vi "AlliGator Overlay Phasor Ratio or Derived Quantity on Source Image v3.vi"(7 "Image Color Scale Information":T2, 8 "Error In":errorcluster, 10 "Source Image Display":T1, 11 "AlliGator IV DVR in":refnum<data-value>) -> (0 "Error Out":errorcluster, 1 "# Overlay Pixels":i32, 2 "Source Image Display out":T1, 3 "AlliGator IV DVR out":refnum<data-value>)   [LabVIEW 2021, in "AlliGator Phasor Plot.lvlib"]
doc: "Computes and overlays the phasor ratio map (or map of a derived quantity) on the Source Image."
uses:
  AlliGator Phasor Plot.lvlib
  <vilib>/vision/Image Controls.llb/IMAQ Image.ctl
  Internal Variables/AlliGator Internal Variables v2.ctl
  Internal Variables/AlliGator Gate Image Set.ctl
  Files/AlliGator FLI Dataset Type.ctl
  Files/AlliGator Data Series Type.ctl
  Dual-Channel Datasets/AlliGator Dataset Channel.ctl
  Settings/AlliGator Gate Arithmetic.ctl
  Source Image/AlliGator Displayed Image.ctl
  Image/Named ROI Description.ctl
  Phasor Graph/AlliGator Decay Metadata v3.ctl
  Decay Analysis/Decay Preprocessing/AlliGator Decay Background Subtraction Info.ctl
  Decay Analysis/Decay Preprocessing/AlliGator Baseline Subtraction Method.ctl
  Graphs/XY Graph/XY Graph Plot Shift Parameters.ctl
  Graphs/XY Graph/XY Graph Plot Shift Method.ctl
  Decay Analysis/Decay Preprocessing/AlliGator Decay Extrapolation Parameters.ctl
  Phasor/Calibration Phasor (m, phi).ctl
  Phasor/Phasor Reference Series.ctl
  Phasor/Phasor Calibration Map v2.ctl
  Phasor/Phasor (g, s).ctl
  Phasor Graph/AlliGator Raw Phasor Plot Data v4.ctl
  Phasor/Phasor Standard Deviation Options.ctl
  AlliGator Phasor Multi-Harmonic Data.ctl
  Phasor/Phasor Harmonic Data.ctl
  Decay Fit Parameter Map/AlliGator Decay Fit Options & Parameters v2.ctl
  Fits/IRF(X)PSED/Decay Fit Options v2.ctl
  Fits/Decay Convolution/Decay Model.ctl
  Fits/Residual Type.ctl
  Fits/IRF(X)PSED/Fit Weights Type.ctl
  Fits/Non-linear Fitting Method v2.ctl
  Fits/Fit Calculation Method.ctl
  Fits/Non-linear Fitting Algorithm.ctl
  Decay Analysis/Decay Fit/AlliGator Decay Fit Parameter Constraints 2.ctl
  Fits/IRF(X)PSED/Decay Fit Parameters In List.ctl
  Fits/IRF(X)PSED/MLE Baseline Offset Type.ctl
  Decay Analysis/Decay Preprocessing/AlliGator Decay Preprocessing Parameters.ctl
  Fits/IRF(X)PSED/Decay Fit Parameters & Derived Quantities List v2.ctl
  Decay Fit Parameter Map/AlliGator Parameter Maps Data.ctl
  Image/Image Color Scale Information.ctl
  Settings/AlliGator Settings List.ctl
  Palette/Image Palette Information.ctl
  Image/Image Display Palette Type.ctl
  Globals, Variables, Constants/AlliGator Variables List.ctl
  Phasor Ratio/AlliGator Phasor Ratio Data.ctl
  Phasor Ratio/AlliGator Phasor Ratio Color-Coded Quantity.ctl
  Phasor/Phasor Ratio Type.ctl
  Settings/AlliGator Partial Data Information.ctl
  Palette/Limit+NaN Colors.ctl
  Variant/Variant to Data/Variant to DBL.vi
  Variant/Variant to Data/Variant to Boolean.vi
  Variant/Variant to Data/Variant to String.vi
  Variant/Variant to Data/Variant to U32.vi
  <vilib>/vision/NI_Vision_Development_Module.lvlib
  Settings/AlliGator Settings.lvlib
  Variant/Variant to Data/Variant to Data.lvlib
  Image/Image.lvlib
  Palette/Palette.lvlib
  Globals, Variables, Constants/AlliGator Globals, Variables & Constants.lvlib
  Phasor Ratio/AlliGator Phasor Ratio.lvlib
  Time/Time.lvlib
  Error/Error.lvlib
  Phasor/Phasor.lvlib
  Utilities/Utilities.lvlib
  Decay Analysis/Decay Preprocessing/AlliGator Decay Preprocessing.lvlib
  Graphs/XY Graph/XY Graph Add-Ons.lvlib
  Phasor Graph/AlliGator Phasor Graph.lvlib
  Files/AlliGator Files.lvlib
  Source Image/AlliGator Source Image.lvlib
  Internal Variables/AlliGator Internal Variables.lvlib
  Fits/Fits.lvlib
  Decay Analysis/Decay Fit/AlliGator Decay Fit.lvlib
  Decay Fit Parameter Map/AlliGator Decay Fit Parameter Map.lvlib
  Dual-Channel Datasets/AlliGator Dual-Channel Datasets.lvlib
panel:
  out "Overlay Copy (s)":dbl
  out "Overlay Erase (s)":dbl
  out "Overlay Compute (s)":dbl
  # "see the AlliGator License on the block diagram (Ctrl+E or Window:Show Block Diagram)"
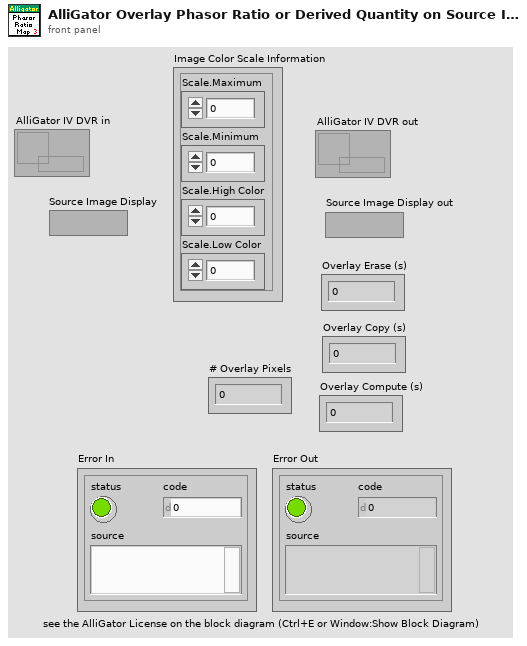
[diagram p1: front panel]
types:
  T1 = typedef "IMAQ Image.ctl" = refnum<image>
  T2 = typedef "Image.lvlib/Image Color Scale Information.ctl" = cluster{"Scale.Maximum":dbl, "Scale.Minimum":dbl, "Scale.High Color":u32, "Scale.Low Color":u32}
  T3 = typedef "Palette.lvlib/Limit+NaN Colors.ctl" = cluster{"Color Scale High Color":cluster{"Red (or Hue) value":u8, "Green (or Sat) value":u8, "Blue (or Light or Val) value":u8}, "Color Scale Low Color":cluster{"Red (or Hue) value":u8, "Green (or Sat) value":u8, "Blue (or Light or Val) value":u8}, "NaN Color":cluster{"Red (or Hue) value":u8, "Green (or Sat) value":u8, "Blue (or Light or Val) value":u8}}
  T4 = typedef "AlliGator Settings.lvlib/AlliGator Settings List.ctl" = enum16{"GUI:Visible Settings Tab", "GUI:Last Run Version", "Source Image:Use Image Histogram for Contrast", "Source Image:Low Count Pixels Rejection Options", "Source Image:High Count Pixels Rejection Options", "Source Image:Use Image Brightness", "Source Image:Blend Overlay with Image Background", "Source Image:Use Fixed ROI Diameter", "Source Image:ROI Diameter", "Source Image:ROI Center Color", "Source Image:Peak Threshold", "Source Image:Intensity Threshold", "Source Image:Image Binning Options", "Source Image:Image Smoothing Options", "Source Image:Image Histogram Active", "Source Image:Invert Binary Mask", "Source Image:Hot Pixel Removal", "Source Image:Overlay Analyzed ROI Center", "Source Image:Auto-Adjust Contrast", "Source Image:Histogram Lower Percentile", "Source Image:Histogram Upper Percentile", "Source Image:Save Source Image", "Source Image:Scale Bar Options", "Source Image:Image Resolution (Pixel Size)", "Source Image:Flatfield Correction", "Source Image:Show Dead Left Columns Correction", "Source Image:Dead Left Columns Correction", "Source Image:Image Pre-Processing Operations Order", "Source Image:Overlay ROI Median", "Source Image:Median Overlay Color", "Data Information:Gate Width", "Data Information:Nanotime Gate Separation", "Data Information:Macrotime Gate Separation", "Data Information:Gate Step", "Data Information:# Gates", "Data Information:Gate Image Exposure", "Data Information:Gate Image Integration", "Data Information:Gates to Skip", "Data Information:Gates to Keep", "Data Information:Define Gates to", "Data Information:Channel Name", "Data Information:Available Channel Names", "Data Information:Channel Arithmetic", "Data Information:Background File Subtraction", "Data Information:Background File", "Data Information:Background Scaling Factor", "Data Information:Background Pile-up Correction", "Data Information:Background Pixel Well Capacity", "Data Information:Laser Period", "Data Information:SYNC Period", "Data Information:Pile-up Correction", "Data Information:Pixel Well Capacity", "Data Information:Dataset Scaling Factor", "Fluorescence Decay_Decay Pre-Processing:Reverse Gates", "Fluorescence Decay_Decay Pre-Processing:Verbose Decay Pre-Processing", "Fluorescence Decay_Decay Pre-Processing:Use Decay Pre-Processing", "Fluorescence Decay_Decay Pre-Processing:Background Subtraction", "Fluorescence Decay_Decay Pre-Processing:Background Definition Range", "Fluorescence Decay_Decay Pre-Processing:Baseline Subtraction Method", "Fluorescence Decay_Decay Pre-Processing:Decay Pre-Processing Operations Order", "Fluorescence Decay_Decay Pre-Processing:Smoothing Parameter", "Fluorescence Decay_Decay Pre-Processing:Shift Decay", "Fluorescence Decay_Decay Pre-Processing:Decay Shift Parameters", "Fluorescence Decay_Decay Pre-Processing:Fold Decay", "Fluorescence Decay_Decay Pre-Processing:# Folds", "Fluorescence Decay_Decay Pre-Processing:1-Normalize Decay", "Fluorescence Decay_Decay Pre-Processing:[0-1]-Normalize Decay", "Fluorescence Decay_Decay Pre-Processing:Smoothen Decay", "Fluorescence Decay_Decay Pre-Processing:Extrapolate Decay", "Fluorescence Decay_Decay Pre-Processing:Use Periodicity", "Fluorescence Decay_Decay Pre-Processing:Use Cursors", "Fluorescence Decay_Decay Pre-Processing:Tail Fraction", "Fluorescence Decay_Decay Pre-Processing:Head Fraction", "Fluorescence Decay_Decay Pre-Processing:Additional Points", "Fluorescence Decay_Decay Pre-Processing:Straighten Decay", "Fluorescence Decay_Decay Pre-Processing:Constant Background", "Fluorescence Decay_Decay Pre-Processing:Pixel-Normalize Decay", "Fluorescence Decay_Advanced Analysis:Extract IRF instead of Decay", "Fluorescence Decay_Advanced Analysis:IRF Extraction Options", "Fluorescence Decay_Advanced Analysis:IRF Optimization Options", "Fluorescence Decay_Advanced Analysis:Square Pulse Options", "Fluorescence Decay_Advanced Analysis:IRF Order", "Fluorescence Decay_Advanced Analysis:IRF Time Constants", "Fluorescence Decay_Advanced Analysis:Wavelet Analysis Options", "Fluorescence Decay_Advanced Analysis:Average Lifetime Options", "Fluorescence Decay_Fit Options:Fit Options", "Fluorescence Decay_Fit Options:Use Legacy Fitting Approach", "Fluorescence Decay_Fit Options:Use Data Information Laser Period", "Fluorescence Decay_Fit Parameters:Displayed Fit Parameters", "Fluorescence Decay_Fit Parameters:Fit Parameter Constraints", "Fluorescence Decay_Fit Parameters:Export Tabulated Results", "Fluorescence Decay_Fit Parameters:MLE Baseline Offset Type", "Fluorescence Decay_Fit Parameters:MLE Baseline Offset", "Fluorescence Decay_Fit Parameters:Guess Parameter Names", "Fluorescence Decay_Fit Parameters:Guess Parameter Values", "Fluorescence Decay_Fit Parameters:Guess Parameters Options", "Fluorescence Decay_Fit Parameters:Optimal Offset Selection Criterion", "Fluorescence Decay_Styles:Show Last Decay Only", "Fluorescence Decay_Styles:Decay Graph Color Array", "Fluorescence Decay:Decay Graph Active", "Fluorescence Decay Statistics:Min Peak Value", "Fluorescence Decay Statistics:Reject Low Decay Peak Pixels", "Fluorescence Decay Statistics:Reject High Decay Peak Pixels", "Fluorescence Decay Statistics:Max Peak Value", "Time Traces:Use File Timestamp", "Time Traces:Time Step", "Time Traces:Use Intensity Correction File", "Time Traces:Intensity Correction File", "Phasor Plot:Phasor Plot Smoothing Options", "Phasor Plot:Phasor Plot Size", "Phasor Plot:Phasor Plot Graphics Options", "Phasor Plot:Cumulative Phasor Plot", "Phasor Plot:Use Phasor Brightness", "Phasor Plot:Blend Overlay with Phasor Background", "Phasor Plot:Save Phasor Plot", "Phasor Plot:Show References", "Phasor Plot:Phasor Ratio Decay Range", "Phasor Plot:Exponential Fading", "Phasor Plot:Phasor Ratio Reference Colors", "Phasor Plot:Reference Radius", "Phasor Plot:Show Color Map Vertices", "Phasor Plot:Phasor Plot Active", "Phasor Plot:Phasor Ratio Color Map Type", "Phasor Plot:Phasor Ratio Color Map", "Phasor Plot:Phasor Ratio Display Range", "Phasor Plot:Selected Image ROI(s)", "Phasor Plot:All Image ROIs", "Phasor Plot:Selected Phasor Plot ROI(s)", "Phasor Plot:All Phasor Plot ROIs", "Phasor Plot:Phasor Ratio Color-Coded Quantity", "Phasor Plot:Store Phasor Harmonics", "Phasor Plot:Draw Reference Segment", "Phasor Plot:User-Defined Quantity", "Phasor Plot:Color Scale High Color", "Phasor Plot:Color Scale Low Color", "Phasor Graph:Phasor Frequency", "Phasor Graph:Phasor Ratio Type", "Phasor Graph:Pixel-level Phasor Computation", "Phasor Graph:Save Phasor Graph", "Phasor Graph:Phasor Graph Active", "Phasor Graph:Phasor SDV Options", "Phasor Calibration:Use Backup Calibration if needed", "Phasor Graph:Define Shortest Lifetime as", "Phasor Calibration:Backup Calibration Type", "Phasor Calibration:Calibration Type", "Phasor Calibration:Calibration Lifetime", "Phasor Calibration:Calibration Map Algorithm", "Single-Exponential Phasor Locus (SEPL):Gate Parameters", "Single-Exponential Phasor Locus (SEPL):User-defined Gate", "Single-Exponential Phasor Locus (SEPL):User-defined IRF", "Single-Exponential Phasor Locus (SEPL):Phasor Parameters", "Single-Exponential Phasor Locus (SEPL):Decay & IRF Parameters", "Single-Exponential Phasor Locus (SEPL):Display Parameters", "Lifetime Analysis:Decay Analysis Parameters", "Lifetime Analysis:Lifetime Map Active", "Plugins:Python Settings", "Miscellaneous:Verbose Mode", "Miscellaneous:Beep after Script", "Miscellaneous:Saved Image File Format", "Miscellaneous:Exported Gate Image Settings", "Miscellaneous:Include Loading in Timing", "Miscellaneous:Verbose Settings Mode", "Miscellaneous:Histogram Options", "Miscellaneous:Beep on Error", "Miscellaneous:# Logical Processors Used", "Miscellaneous:ROI Description Max Characters", "Miscellaneous:Verbose Error Mode", "Miscellaneous:Transparent Mask Color"}
  T5 = typedef "AlliGator Settings.lvlib/AlliGator Partial Data Information.ctl" = cluster{"Laser Period":dbl[unit], "SYNC Period":dbl[unit], "# Gates":u32, "Gate Separation":dbl[unit]}
  T6 = typedef "Phasor.lvlib/Phasor Ratio Type.ctl" = enum32{"Intensity-weighted", "Amplitude-weighted"}
  T7 = typedef "AlliGator Phasor Ratio.lvlib/AlliGator Phasor Ratio Color-Coded Quantity.ctl" = enum16{"Phasor Ratio (f1 or a1)", "Average Lifetime (<tau>_i or <tau>_a))", "User-Defined Quantity"}
  T8 = typedef "AlliGator Phasor Ratio.lvlib/AlliGator Phasor Ratio Data.ctl" = cluster{"Complex Phasor":csg, "Phasor Ratio":sgl, "z_1":csg, "z_2":csg, "Mapped Quantity":sgl}
  T9 = typedef "AlliGator Globals, Variables & Constants.lvlib/AlliGator Variables List.ctl" = enum16{"---- GUI ----", "GUI:Initialization Status", "GUI:State Indicators Refnum", "GUI:Original AlliGator Menu Items", "GUI:Current Action Loop State", "GUI:Script in progress", "GUI:Playback", "GUI:Loop Playback", "GUI:Search ROI Used", "GUI:Search ROI", "Decay Graph Max Legend Size", "Intensity Graph Max Legend Size", "Decay Statistics Graph Max Legend Size", "Phasor Graph Max Legend Size", "Phasor Ratio Graph Max Legend Size", "Lifetime Graph Max Legend Size", "---- Files ----", "Files:Export Dataset Frames as Individual Files", "Files:Show Batch Export Help Balloons", "Files:Frames in Dataset", "Files:ptu File Frame Start Indices", "Files:Current Frame in Dataset", "Files:Current Frame Timestamp", "Files:Dataset Loaded", "Files:Dataset Metadata", "Files:Dataset Channel", "Files:Dataset Data Description", "Files:Background Dataset Metadata", "Files:Background Dataset Channel", "Files:Background Dataset Data Description", "Files:Background File Subtraction", "Files:Background File Path", "Files:Background File Pile-up Correction", "Files:Background File Pixel Well Capacity", "Files:Background File Scaling Factor", "Files:Current Dataset Load Settings", "Files:Dataset Path", "Files:ICCD-specific Information", "Files:Macrotime Gate Separation", "------ Python Plugins ------", "Python Plugins:Information", "Python Plugins:Python Session", "Python Plugins:Valid Python Session?", "---- Source Image ----", "Source Image:ROIs", "Source Image:Current ROI", "Source Image:ROI Event Refnum", "X_Source Image:Display Range", "X_Source Image:Palette Information", "X_Source Image:Type of Displayed Image", "X_Time Gate Slider", "Source Image:Palette List", "Source Image:Scale", "Source Image:ROI Overlay Color", "Source Image:Overlay to Erase", "Source Image:Is Displayed Image Accumulated", "Source Image:White Light Image Modified", "Source Image:Mask Image Modified", "---- Image Profile Window ----", "Image Profile:Window Event Refnum", "Image Profile:IntensityType", "Image Profile:Intensity Average Type", "Image Profile:Intensity-weighted SDV", "Image Profile:Box Profile Type", "Image Profile:Window Open", "Image Profile:Plotted Fit Parameter", "------ Phasor Graph -------", "Phasor Graph:Show Line", "---- Phasor Plot ---", "Phasor Plot:Parameters Changed", "Phasor Plot:FLI Dataset Modified since last Calculation", "Phasor Harmonics Data", "Selected Phasor Harmonics", "Phasor Harmonic Manager Event Refnum", "Phasor Plot:ROIs", "Phasor Plot:Current ROI", "Phasor Plot:ROI Event Refnum", "Phasor Plot:Image Reference Points", "Phasor Plot:Computed", "Phasor Plot:Palette Information", "Phasor Plot:Palette List", "Phasor Plot:Phasor Ratio Palette Information", "Phasor Plot:Phasor Ratio Palette List", "Phasor Plot:Image Scale", "Phasor Plot:Image Overlay to Erase", "Phasor Plot:Image Elements to Update", "Phasor Plot:Current Calculation Parameters", "Phasor Plot:Current Calibration Options", "Phasor Plot:Reset Cumulated Phasor Plot", "Phasor Plot:Reference 1", "Phasor Plot:Lifetime Reference 1", "Phasor Plot:Reference 1 Frequency", "Phasor Plot:Reference 2", "Phasor Plot:Lifetime Reference 2", "Phasor Plot:Reference 2 Frequency", "---- Decay Analysis ----", "Number of Selected Decays to Fit", "LS Fit Results", "LAR Fit Results", "BS Fit Results", "Last Decay Max - Min", "Best Fit Parameters", "Best Fit Parameter Names", "Actual Size X", "Actual Size Y", "Binning X", "Binning Y", "Actual # Gates", "Dataset Number", "Gates to...", "Gates Skipped", "Gates to keep", "Gate Step", "Gate Separation", "Reversed Gates", "Pile-up Correction", "Pixel Well Capacity", "Background Subtracted", "Background Subtraction Method", "Background Definition Range", "Background File (deprecated)", "Number of Dataset Accumulated", "Array of Accumulated Dataset Paths", "Do Averaged Datasets", "Destination File Path", "Process Plot Target", "Use 1/D as Phasor Frequency", "---- Decay Fit Parameter Map -----", "Decay Fit Parameter Map:Palette Information", "Decay Fit Parameter Map:Palette List", "Decay Fit Parameter Map:X Resolution", "Decay Fit Parameter Map:Y Resolution", "---- Parameter Map ----", "Parameter Map:Palette Information", "Parameter Map:Palette List", "------- Local Decay Window ---------", "Local Decay Graph Window:Event Refnum", "Local Decay Graph Window:Use normalized IRF for convolution", "----- Miscellaneous ----", "Misc:Skippable Dialog Windows Status"}
  T10 = typedef "Palette.lvlib/Image Palette Information.ctl" = cluster{"Palette Name [# Colors,int?,inv?]":string, "Palette Type":T11, "Palette Colors":u32[], "Interpolate?":bool}
  T11 = typedef "Image.lvlib/Image Display Palette Type.ctl" = u32
  T12 = enum32{"Interpolate Reference Colors", "Use Custom Map"}
  T13 = cluster{"Reference 1":u32, "Reference 2":u32, "Boundary":u32}
  T14 = typedef "Phasor.lvlib/Phasor (g, s).ctl" = cluster{"g":dbl, "s":dbl}
  T15 = cluster{"Red (or Hue) value":u8, "Green (or Sat) value":u8, "Blue (or Light or Val) value":u8}
  T16 = cluster{"Red (or Hue) value":u8, "Green (or Sat) value":u8, "Blue (or Light or Val) value":u8}[]
  T17 = typedef "AlliGator Internal Variables.lvlib/AlliGator Internal Variables v2.ctl" = cluster{"Displayed Image":T1, "White Light Image":T1, "Mask Image":T1, "ROI Mask Image":T1, "Current Dataset Images 1":T18, "Background Dataset Images 1":T18, "Current Dataset Images 2":T18, "Background Dataset Images 2":T18, "Current Dataset Arithmetic Images":T18, "Accumulated Dataset Images 1":T18, "Accumulated Dataset Images 2":T18, "Accumulated Dataset Arithmetic Images":T18, "Phasor Plot Image":T1, "Decay Fit Parameter Map Image":T1, "Parameter Map Image":T1, "Single Data Point Path":path, "White Light Image Path":path, "Mask Image Path":path, "Time-Series Folder":path, "[Time-Series Paths]":path[], "Current Dataset":i32, "Single Dataset Type":T19, "Current Folder":string, "AlliGator Data Series Type":T20, "# Datasets":i32, "Dual-Channel Dataset":bool, "Selected Channel Name":string, "Dataset Channel":T21, "Channel Arithmetic":T22, "Dual-Channel Background Dataset":bool, "Background Channel":T21, "Dual-Channel Accumulated Dataset":bool, "Start Time":dbl, "[Time-Series Timestamps]":dbl[], "[Intensity Corrections]":dbl[], "Time Series Script":bool, "Type of Displayed Image":T23, "Gate Image Slide":u16, "# Gates":i32, "ROIs":T24[], "ROI Decay":cluster{"t Array":dbl[], "I Array":dbl[]}, "Valid Decay":bool, "Decay  Metadata":T26, "Reference Decay Plot Name":string, "Reference Decay":cluster{"t Array":dbl[], "I Array":dbl[]}, "Decay Shift Plot":cluster{"Time Stamps":dbl[], "Decay Shifts":dbl[]}, "[Decays Max Values]":sgl[], "[Decays Min Values]":sgl[], "Calibration Phasor":T32, "Calibration Phasor Series":T33, "Phasor Calibration Map":T34, "Calibration Map MD5 Digest":string, "Last Raw Phasor":T14, "Last Calibrated Phasor":T14, "Last Calibrated Phasor SDV":T14, "Phasor Graph:Phasor Plot":cluster{"g Array":dbl[], "s Array":dbl[]}, "Phasor Graph:Phasor SDV Plot":cluster{"g Array":dbl[], "s Array":dbl[]}, "[Phasor Graph:Raw Phasor Plots]":T35[], "Phasor Plot locked to Ref 1":i32, "[Phasor Plot(s) locked to Ref 1]":i32[], "[Phasor Plot(s) locked to Ref 2]":i32[], "[Pixel Phasors]":T14[], "[[Sum Image]]":dbl[][], "[[CSG Phasors]]":csg[][], "[[Valid Pixel?]]":bool[][], "I/m/phi Dataset":cluster{"I/m/phi Dataset?":bool, "Base Frequency":dbl[unit], "Harmonic Orders":u8[]}, "Multi Phasor Plot Data":T37, "Decay Fit Options & Parameters":T39, "Fit Options: Decay Preprocessing Parameters":T50, "Fit Options: Reference Decay":cluster{"t Array":dbl[], "I Array":dbl[]}, "Is Full Image Parameters Map":bool, "Is Single-Pixels Parameters Map":bool, "NLSF Parameters Map X Resolution":i32, "NLSF Parameters Map Y Resolution":i32, "[Single Decay Fit Parameters]":dbl[], "Fit Model":T41, "[[Multiple Decays Fit Parameters]]":dbl[][], "[[Multiple Decays Fit Parameter SDVs]]":dbl[][], "[[IRFs]]":dbl[][], "IRF Array Time Axis":dbl[], "Decay Array Time Axis":dbl[], "[Decay Fit Parameter Names]":T51[], "[[Phasor Ratios]]":dbl[][], "[[Average Lifetimes]]":dbl[][], "Amplitude Weighted Average Lifetime":bool, "[Decay Sum]":dbl[], "[Map Set Names]":string[], "[Parameter Maps]":T52[], "[[User-defined Quantities]]":dbl[][], "User-defined Quantity":string}
  T18 = typedef "AlliGator Internal Variables.lvlib/AlliGator Gate Image Set.ctl" = cluster{"SGL Image Max":T1, "SGL Image Sum":T1, "SGL Gate Images":T1[], "SGL Image Min":T1}
  T19 = typedef "AlliGator Files.lvlib/AlliGator FLI Dataset Type.ctl" = enum16{"HDF5 FLI Dataset", "Gate Image Folder", ".sdt FLI Dataset (Becker & Hickl)", ".ptu FLI Dataset (PicoQuant)", "SS1 FLI Dataset", "SS2 FLI Dataset", "I/m/phi Dataset", ".bin FLI Dataset (PicoQuant Binned)", ".bin FLI Dataset (Piccolo Binned)", ".mat FLI Dataset"}
  T20 = typedef "AlliGator Files.lvlib/AlliGator Data Series Type.ctl" = enum16{"Not a Supported Series", "Gate Images Folder Series", "SwissSPAD 2 Dataset Series", "B&H FLI Dataset Series", "PicoQuant PTU FLI Dataset Series", "PicoQuant BIN FLI Dataset Series", "Piccolo hist BIN FLI Dataset Series", "HDF5 FLI Dataset Series"}
  T21 = typedef "AlliGator Dual-Channel Datasets.lvlib/AlliGator Dataset Channel.ctl" = enum16{"G2", "INT"}
  T22 = typedef "AlliGator Settings.lvlib/AlliGator Gate Arithmetic.ctl" = enum16{"None", "INT-G2", "G2/INT*<INT>", "(1 - G2/INT)*<INT>"}
  T23 = typedef "AlliGator Source Image.lvlib/AlliGator Displayed Image.ctl" = enum16{"Single Gate", "Sum of All Gates", "Max of All Gates", "Min of All Gates", "-", "White Ligth Image", "Mask Image"}
  T24 = typedef "Image.lvlib/Named ROI Description.ctl" = cluster{"ROI Descriptor":T25, "ROI Name":string, "Overlay Color":u32}
  T25 = typedef "ROI Descriptor" = cluster{"Global Rectangle":i32[], "Contours":cluster{"ID":enum32{"External", "Internal"}, "Type":u32, "Coordinates":i32[]}[]}
  T26 = typedef "AlliGator Phasor Graph.lvlib/AlliGator Decay Metadata v3.ctl" = cluster{"ROI Descriptor":T25, "ROI Center":cluster{"X":i32, "Y":i32}, "Decay Background Subtraction Info":T27, "Decay Reverted":bool, "Decay Smoothened":bool, "Decay Straightened":bool, "Fitted Tau (Decay Straightening)":dbl, "Decay Shift Parameters":T29, "Decay Shifted":bool, "Decay Extrapolated":bool, "Decay Extrapolation Parameters":T31, "Decay Normalized":bool, "Fold Decay":bool, "# Folds":u32}
  T27 = typedef "AlliGator Decay Preprocessing.lvlib/AlliGator Decay Background Subtraction Info.ctl" = cluster{"Laser Period":dbl[unit], "Gate Duration":dbl[unit], "Baseline Subtraction Method":T28, "Background Definition Range":cluster{"Min Gate":dbl[unit], "Max Gate":dbl[unit]}, "Total Intensity w/o Bkgd Subtraction":dbl, "Bkgd-subtracted Intensity (exp)":dbl, "# Data Points":i32, "Background/Gate":dbl, "Fitted Lifetime":dbl[unit], "Bkgd-subtracted Intensity (theo)":dbl}
  T28 = typedef "AlliGator Decay Preprocessing.lvlib/AlliGator Baseline Subtraction Method.ctl" = enum16{"Mean", "Min", "Square Gated Single-Exponential", "File", "Constant"}
  T29 = typedef "XY Graph Add-Ons.lvlib/XY Graph Plot Shift Parameters.ctl" = cluster{"Type":T30, "Shift":dbl[unit], "Threshold":dbl, "Rotate":bool}
  T30 = typedef "XY Graph Add-Ons.lvlib/XY Graph Plot Shift Method.ctl" = enum16{"Default", "CFD", "Threshold", "Cross-Correlation"}
  T31 = typedef "AlliGator Decay Preprocessing.lvlib/AlliGator Decay Extrapolation Parameters.ctl" = cluster{"Additional Points":u32, "Head Fraction":dbl, "Fitted Tau":dbl, "Use Periodicity":bool, "Use Cursors":bool, "Tail Fraction":dbl}
  T32 = typedef "Phasor.lvlib/Calibration Phasor (m, phi).ctl" = cluster{"m":dbl, "phi":dbl, "Phasor Frequency":dbl[unit], "Reference Lifetime":dbl[unit]}
  T33 = typedef "Phasor.lvlib/Phasor Reference Series.ctl" = cluster{"m Array":dbl[], "phi Array":dbl[], "Phasor Frequency":dbl[unit], "Calibration Lifetime":dbl[unit]}
  T34 = typedef "Phasor.lvlib/Phasor Calibration Map v2.ctl" = cluster{"Phasor Frequency":dbl[unit], "Calibration Lifetime":dbl[unit], "ROI Centers":cluster{"X":i32, "Y":i32}[], "ROI Descriptors":T25[], "Map Resolution X":i32, "Map Resolution Y":i32, "z Array":cdb[]}
  T35 = typedef "AlliGator Phasor Graph.lvlib/AlliGator Raw Phasor Plot Data v4.ctl" = cluster{"Phasor Plot Name":string, "Raw Phasor Plot":T14[], "Phasor Frequency":dbl[unit], "[Decay Metadata]":T26[], "Raw Phasor Plot SDV":T14[], "Phasor SDV Options":T36, "[Calibration Phasor]":T32[]}
  T36 = typedef "Phasor.lvlib/Phasor Standard Deviation Options.ctl" = cluster{"Compute Estimated SDV":bool, "# Replicas":u32, "Use Estimated Average Phasor":bool}
  T37 = typedef "AlliGator Phasor Plot.lvlib/AlliGator Phasor Multi-Harmonic Data.ctl" = cluster{"Base Frequency":dbl[unit], "# Harmonics":u8, "Harmonic Orders":u8[], "Phasor Plot Settings Checksum":u64, "Phasor Harmonic Data Array":T38[]}
  T38 = typedef "Phasor.lvlib/Phasor Harmonic Data.ctl" = cluster{"Phasor Harmonic Name":string, "Phasor Plot Settings Checksum":u64, "Phasor Frequency":dbl[unit], "Base Frequency":dbl[unit], "Harmonic Order":u8, "Phasor Plot Parameters":string, "Phasor Array [[CSG]]":csg[][], "Dataset File Path":path}
  T39 = typedef "AlliGator Decay Fit Parameter Map.lvlib/AlliGator Decay Fit Options & Parameters v2.ctl" = cluster{"SYNC Period":dbl[unit], "Fit Options":T40, "Fit Parameter Constraints":T47[], "MLE Baseline Offset":dbl, "MLE Baseline Offset Type":T49}
  T40 = typedef "Fits.lvlib/Decay Fit Options v2.ctl" = cluster{"Show Fit Residuals":bool, "Fit Model":T41, "Residual Type":T42, "Max Decay Percentile":dbl, "Min Decay Percentile":dbl, "Show Full Decay":bool, "Weights":T43, "Fitting Method":T44, "Compute Parameter Uncertainties":bool, "Periodic Boundaries":bool, "Model Calculation":T45, "Period":dbl[unit], "Termination Criteria":cluster{"Max Iterations":i32, "Max Function Calls":i32, "Max Time":dbl[unit], "Function Tolerance":dbl, "Parameter Tolerance":dbl, "Gradient Tolerance":dbl, "Min Lambda":dbl, "Max Lambda":dbl, "Initial Tick Count":u32}, "Offset Resolution":dbl[unit], "Use Local IRF":bool, "Fitting Algorithm":T46}
  T41 = typedef "Fits.lvlib/Decay Model.ctl" = enum16{"1-Exponential", "2-Exponentials"}
  T42 = typedef "Fits.lvlib/Residual Type.ctl" = enum16{"Standard", "Normalized", "Reduced"}
  T43 = typedef "Fits.lvlib/Fit Weights Type.ctl" = enum16{"Unweighted", "1/Variance", "Best of All"}
  T44 = typedef "Fits.lvlib/Non-linear Fitting Method v2.ctl" = enum16{"Least Square", "Least Absolute Residual", "Bisquare", "MLE", "-", "Best of All"}
  T45 = typedef "Fits.lvlib/Fit Calculation Method.ctl" = enum16{"Simulation", "Convolution", "Integration"}
  T46 = typedef "Fits.lvlib/Non-linear Fitting Algorithm.ctl" = enum16{"Levenberg-Marquardt", "Trust-Region Dogleg"}
  T47 = typedef "AlliGator Decay Fit.lvlib/AlliGator Decay Fit Parameter Constraints 2.ctl" = cluster{"Fit Parameter":T48, "Min Value":dbl, "Max Value":dbl, "Global":bool, "Used":bool}
  T48 = typedef "Fits.lvlib/Decay Fit Parameters In List.ctl" = enum16{"Offset", "Baseline", "A_1", "tau_1", "A_2", "tau_2"}
  T49 = typedef "Fits.lvlib/MLE Baseline Offset Type.ctl" = enum32{"Absolute", "Percentage"}
  T50 = typedef "AlliGator Decay Preprocessing.lvlib/AlliGator Decay Preprocessing Parameters.ctl" = cluster{"Background Subtraction":bool, "Straighten Decay":bool, "Reverse Gates":bool, "1-Normalized Decay":bool, "Smoothen Decay":bool, "Smoothing Parameter":dbl, "Shift Decay":bool, "Decay Shift Parameters":T29, "Extrapolate Decay":bool, "Additional Points":u32, "Head Fraction":dbl, "Pixel-Normalize Decay":bool, "Use Periodicity":bool, "Use Cursors":bool, "Tail Fraction":dbl, "Use Decay Pre-Processing":bool, "Fold Decay":bool, "# Folds":u32, "[0-1]-Normalized Decay":bool}
  T51 = typedef "Fits.lvlib/Decay Fit Parameters & Derived Quantities List v2.ctl" = enum16{"Offset", "Baseline", "A_1", "tau_1", "A_2", "tau_2", "<tau>_a", "f1_a", "f2_a", "<tau>_i", "f1_i", "f2_i", "-", "R^2", "Chi^2"}
  T52 = typedef "AlliGator Decay Fit Parameter Map.lvlib/AlliGator Parameter Maps Data.ctl" = cluster{"Map Set Name":string, "[Parameter Names]":string[], "[[Parameters]]":dbl[][], "[[Parameter SDVs]]":dbl[][], "Decay Array Time Axis":dbl[], "[[IRFs]]":dbl[][], "IRF Array Time Axis":dbl[]}
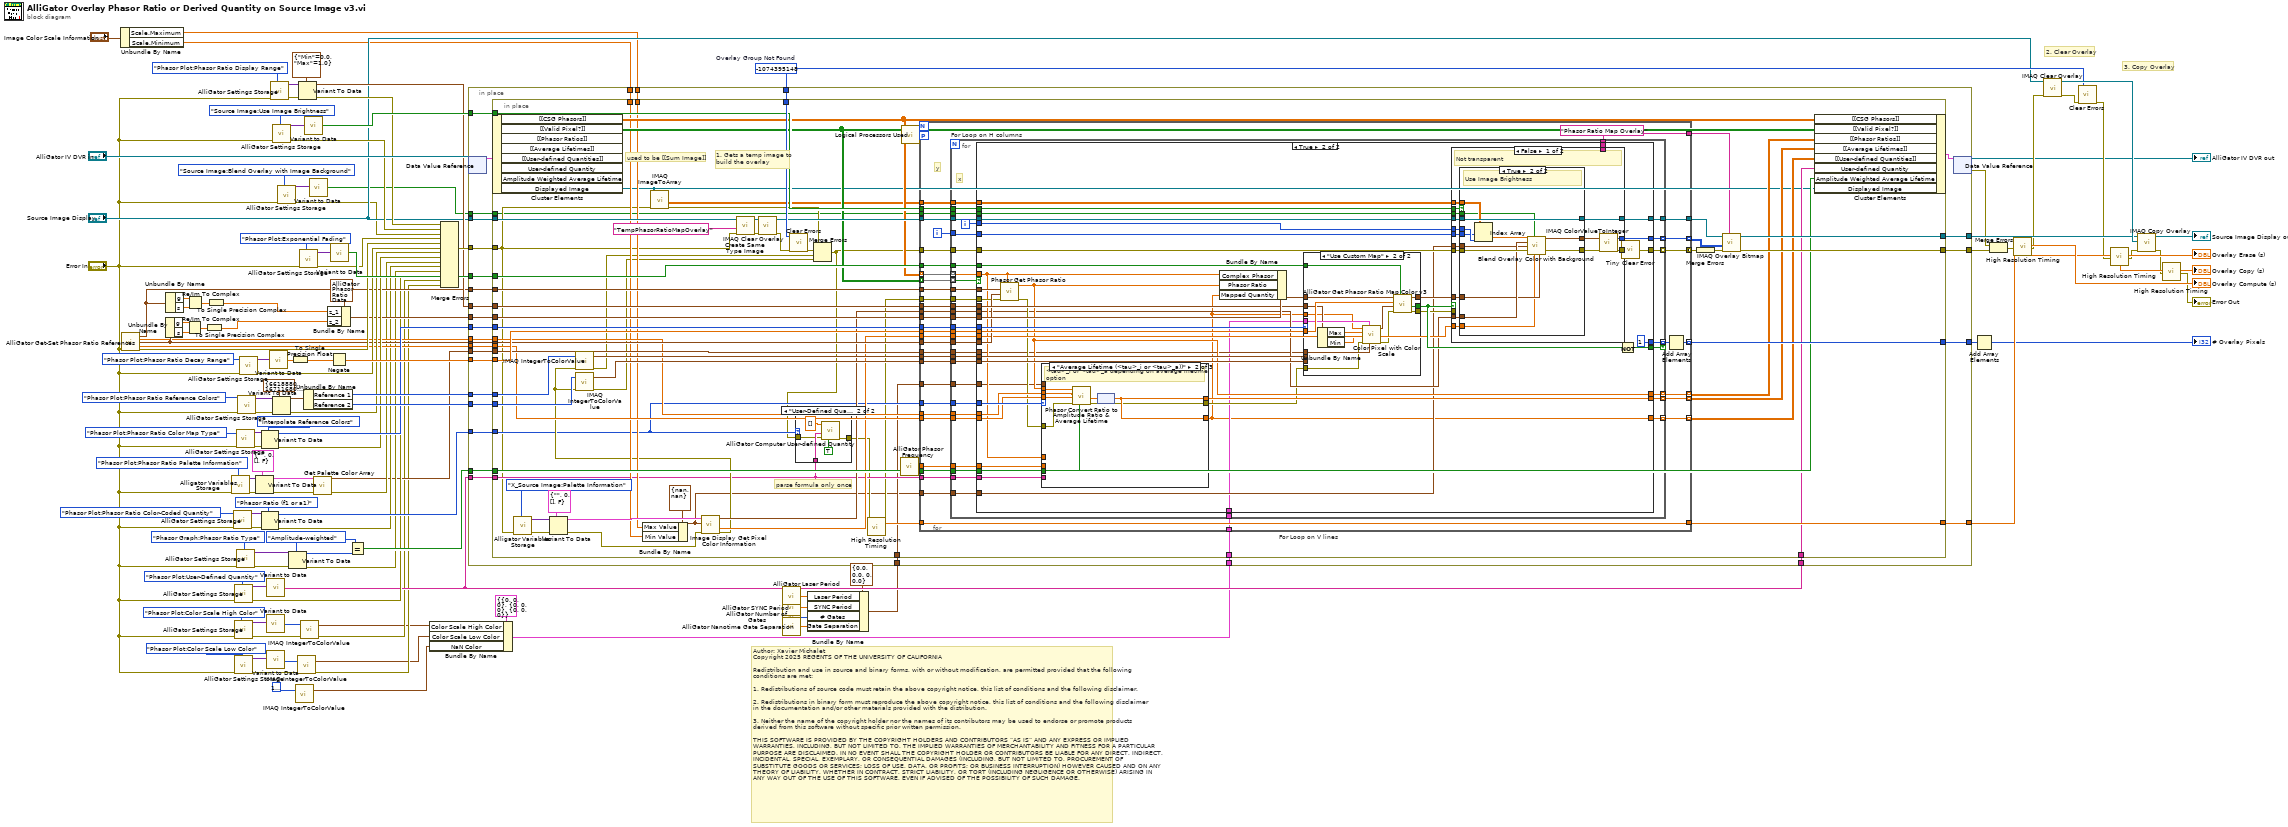
[diagram p0: block diagram]
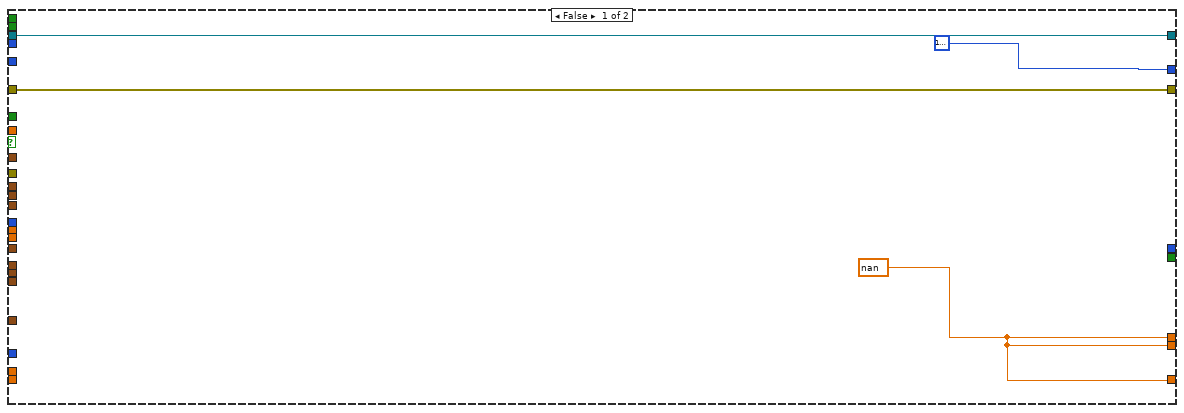
[diagram p2: hidden frame]
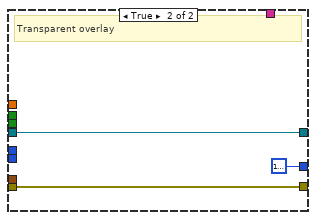
[diagram p4: hidden frame]
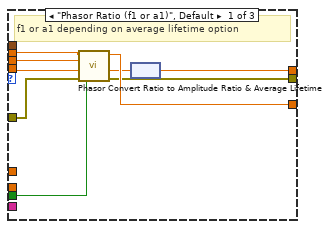
[diagram p5: hidden frame]
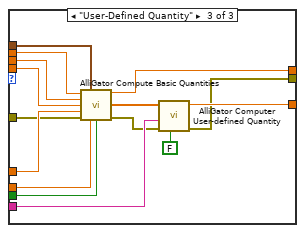
[diagram p6: hidden frame]
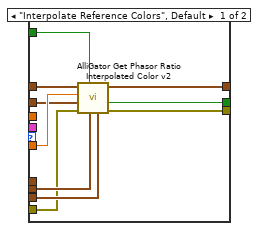
[diagram p7: hidden frame]
diagram:
  w46 = Phasor_Ratio_Type."Amplitude-weighted" ("Phasor Ratio Type")
  w104 = -1074395148  # Overlay Group Not Found
  # "Author: Xavier Michalet\nCopyright 2025 REGENTS OF THE UNIVERSITY OF CALIFORNIA\n\nRedistribution and use in source and binary forms, with or without modification, are permitted provided that the following conditions are met:\n\n1. Redistributions of source code must retain the above copyright notice, this list of conditions and the following disclaimer.\n\n2. Redistributions in binary form must reproduce the above copyright notice, this list of conditions and the following disclaimer in the documentation and/or other materials provided with the distribution.\n\n3. Neither the name of the copyright holder nor the names of its contributors may be used to endorse or promote products derived from this software without specific prior written permission.\n\nTHIS SOFTWARE IS PROVIDED BY THE COPYRIGHT HOLDERS AND CONTRIBUTORS “AS IS” AND ANY EXPRESS OR IMPLIED WARRANTIES, INCLUDING, BUT NOT LIMITED TO, THE IMPLIED WARRANTIES OF MERCHANTABILITY AND FITNESS FOR A PARTICULAR PURPOSE ARE DISCLAIMED. IN NO EVENT SHALL THE COPYRIGHT HOLDER OR CONTRIBUTORS BE LIABLE FOR ANY DIRECT, INDIRECT, INCIDENTAL, SPECIAL, EXEMPLARY, OR CONSEQUENTIAL DAMAGES (INCLUDING, BUT NOT LIMITED TO, PROCUREMENT OF SUBSTITUTE GOODS OR SERVICES; LOSS OF USE, DATA, OR PROFITS; OR BUSINESS INTERRUPTION) HOWEVER CAUSED AND ON ANY THEORY OF LIABILITY, WHETHER IN CONTRACT, STRICT LIABILITY, OR TORT (INCLUDING NEGLIGENCE OR OTHERWISE) ARISING IN ANY WAY OUT OF THE USE OF THIS SOFTWARE, EVEN IF ADVISED OF THE POSSIBILITY OF SUCH DAMAGE."
  # "3. Copy Overlay"
  # "2. Clear Overlay"
  n1 = Unbundle By Name("Image Color Scale Information") -> ("Scale.Maximum"=w38:dbl, "Scale.Minimum"=w37:dbl)
  n2 = call "AlliGator Get-Set Phasor Ratio References.vi"("error in (no error)"="Error In") -> ("Reference Phasor 1"=w54:T14, "Reference Lifetime 1"=w50:dbl[unit], "Reference Phasor 2"=w53:T14, "Reference Lifetime 2"=w49:dbl[unit], "error out"=w88:errorcluster)  [unwired: 7 in, 3 out]
  n3 = Unbundle By Name(w53) -> ("g"=w120:dbl, "s"=w121:dbl)
  n4 = Unbundle By Name(w54) -> ("g"=w129:dbl, "s"=w128:dbl)
  n5 = Re/Im To Complex(1:w121, 2:w120) -> (0:w122:cdb)
  n6 = Re/Im To Complex(1:w128, 2:w129) -> (0:w127:cdb)
  n7 = To Single Precision Complex(1:w122) -> (0:w52:csg)
  n8 = To Single Precision Complex(1:w127) -> (0:w60:csg)
  n9 = call "Alligator Variables Storage.vi"("AlliGator Variable"=AlliGator_Variables_List."Phasor Plot:Phasor Ratio Palette Information" ("Alligator Variable"), "Error In"="Error In") -> ("Error Out"=w92:errorcluster, "Data out"=w93:variant)  [unwired: 7 in, 1 out]
  n10 = call "AlliGator Settings Storage.vi"("AlliGator Settings List"=AlliGator_Settings_List."Phasor Plot:Phasor Ratio Color-Coded Quantity", "Error In"="Error In") -> ("Error Out"=w58:errorcluster, "Variant Data out"=w57:variant)  [unwired: 8 in]
  n11 = call "AlliGator Settings Storage.vi"("AlliGator Settings List"=AlliGator_Settings_List."Phasor Plot:Color Scale High Color", "Error In"="Error In") -> ("Error Out"=w9:errorcluster, "Variant Data out"=w17:variant)  [unwired: 8 in]
  n12 = call "AlliGator Settings Storage.vi"("AlliGator Settings List"=AlliGator_Settings_List."Phasor Plot:User-Defined Quantity", "Error In"="Error In") -> ("Error Out"=w34:errorcluster, "Variant Data out"=w35:variant)  [unwired: 8 in]
  n13 = call "AlliGator Settings Storage.vi"("AlliGator Settings List"=AlliGator_Settings_List."Phasor Plot:Color Scale Low Color", "Error In"="Error In") -> ("Error Out"=w11:errorcluster, "Variant Data out"=w15:variant)  [unwired: 8 in]
  n14 = call "AlliGator Settings Storage.vi"("AlliGator Settings List"=AlliGator_Settings_List."Phasor Plot:Phasor Ratio Color Map Type", "Error In"="Error In") -> ("Error Out"=w97:errorcluster, "Variant Data out"=w98:variant)  [unwired: 8 in]
  n15 = call "AlliGator Settings Storage.vi"("AlliGator Settings List"=AlliGator_Settings_List."Phasor Graph:Phasor Ratio Type", "Error In"="Error In") -> ("Error Out"=w44:errorcluster, "Variant Data out"=w45:variant)  [unwired: 8 in]
  n16 = call "AlliGator Settings Storage.vi"("AlliGator Settings List"=AlliGator_Settings_List."Phasor Plot:Phasor Ratio Reference Colors", "Error In"="Error In") -> ("Error Out"=w99:errorcluster, "Variant Data out"=w117:variant)  [unwired: 8 in]
  n17 = call "AlliGator Settings Storage.vi"("AlliGator Settings List"=AlliGator_Settings_List."Phasor Plot:Phasor Ratio Decay Range", "Error In"="Error In") -> ("Error Out"=w87:errorcluster, "Variant Data out"=w125:variant)  [unwired: 8 in]
  n18 = Variant To Data(error in=w92, type=T10 {"Palette Name [# Colors,int?,inv?]"="", "Palette Type"=0, "Palette Colors"=[], "Interpolate?"=FALSE} ("Image Display Palette Information"), Variant=w93) -> (data=w21:T10, error out=w20:errorcluster)
  n19 = Variant To Data(error in=w97, type=T12."Interpolate Reference Colors" ("Phasor Ratio Color Map Type"), Variant=w98) -> (data=w95:T12, error out=w85:errorcluster)
  n20 = Variant To Data(error in=w58, type=AlliGator_Phasor_Ratio_Color-Coded_Quantity."Phasor Ratio (f1 or a1)" ("Displayed Quantity"), Variant=w57) -> (data=w51:T7, error out=w42:errorcluster)
  n21 = call-poly "Variant to Data.vi"("Variant"=w17) -> ("Value"=w13:u32)  [unwired: 8 in]
  n22 = call-poly "Variant to Data.vi"("Variant"=w35) -> ("String"=w32:string)  [unwired: 8 in]
  n23 = call-poly "Variant to Data.vi"("Variant"=w15) -> ("Value"=w12:u32)  [unwired: 8 in]
  n24 = call-poly "Variant to Data.vi"("Variant"=w125) -> ("Value"=w124:dbl)  [unwired: 8 in]
  n25 = call "AlliGator Settings Storage.vi"("AlliGator Settings List"=AlliGator_Settings_List."Phasor Plot:Phasor Ratio Display Range", "Error In"="Error In") -> ("Error Out"=w66:errorcluster, "Variant Data out"=w64:variant)  [unwired: 8 in]
  n26 = Variant To Data(error in=w99, type=T13 {"Reference 1"=6618880, "Reference 2"=16711680, "Boundary"=16776960} ("Phasor Ratio Reference Colors"), Variant=w117) -> (data=w115:T13, error out=w86:errorcluster)
  n27 = call "AlliGator Settings Storage.vi"("AlliGator Settings List"=AlliGator_Settings_List."Source Image:Use Image Brightness", "Error In"="Error In") -> ("Error Out"=w68:errorcluster, "Variant Data out"=w103:variant)  [unwired: 8 in]
  n28 = call "AlliGator Settings Storage.vi"("AlliGator Settings List"=AlliGator_Settings_List."Source Image:Blend Overlay with Image Background", "Error In"="Error In") -> ("Error Out"=w23:errorcluster, "Variant Data out"=w25:variant)  [unwired: 8 in]
  n29 = Variant To Data(error in=w44, type=w46, Variant=w45) -> (data=w47:T6, error out=w33:errorcluster)
  n30 = To Single Precision Float(number=w124) -> (single precision float=w123:sgl)
  n31 = call "IMAQ IntegerToColorValue"("U32 value"=u32 16777216) -> ("Color Value"=w4:T15)  [unwired: 4 in, 3 out]
  n32 = call "IMAQ IntegerToColorValue"("error in (no error)"=w11, "U32 value"=w12) -> ("error out"=w10:errorcluster, "Color Value"=w5:T15)  [unwired: 3 in, 2 out]
  n33 = Variant To Data(error in=w66, type=cluster{"Min":dbl, "Max":dbl} {"Min"=0.0, "Max"=1.0} ("Phasor Ratio Display Range"), Variant=w64) -> (data=w55:cluster{"Min":dbl, "Max":dbl}, error out=w65:errorcluster)
  n34 = call "AlliGator Settings Storage.vi"("AlliGator Settings List"=AlliGator_Settings_List."Phasor Plot:Exponential Fading", "Error In"="Error In") -> ("Error Out"=w89:errorcluster, "Variant Data out"=w111:variant)  [unwired: 8 in]
  n35 = call "IMAQ IntegerToColorValue"("error in (no error)"=w9, "U32 value"=w13) -> ("error out"=w8:errorcluster, "Color Value"=w6:T15)  [unwired: 3 in, 2 out]
  n36 = Unbundle By Name(w115) -> ("Reference 1"=w114:u32, "Reference 2"=w113:u32)
  n37 = call-poly "Variant to Data.vi"("Variant"=w103) -> ("Value"=w101:bool)  [unwired: 8 in]
  n38 = call-poly "Variant to Data.vi"("Variant"=w25) -> ("Value"=w22:bool)  [unwired: 8 in]
  n39 = call "Get Palette Color Array.vi"("error in (no error)"=w20, "Image Display Palette Information"=w21) -> ("error out"=w19:errorcluster, "1D Color value array"=w18:T16)  [unwired: 8 in]
  n40 = Bundle By Name(cluster=T8 {"Complex Phasor"=0.0+0.0i, "Phasor Ratio"=0.0, "z_1"=0.0+0.0i, "z_2"=0.0+0.0i, "Mapped Quantity"=0.0} ("Phasor Ratio Data"), "z_1"=w60, "z_2"=w52) -> (w61:T8)
  n41 = Negate(x=w123) -> (-x=w119:sgl)
  n42 = call-poly "Variant to Data.vi"("Variant"=w111) -> ("Value"=w110:bool)  [unwired: 8 in]
  n43 = Equal?(x=w46, y=w47) -> (x = y?=w43:bool)
  n44 = Bundle By Name(cluster=T3 {"Color Scale High Color"={"Red (or Hue) value"=0, "Green (or Sat) value"=0, "Blue (or Light or Val) value"=0}, "Color Scale Low Color"={"Red (or Hue) value"=0, "Green (or Sat) value"=0, "Blue (or Light or Val) value"=0}, "NaN Color"={"Red (or Hue) value"=0, "Green (or Sat) value"=0, "Blue (or Light or Val) value"=0}} ("Limit Colors"), "Color Scale High Color"=w6, "Color Scale Low Color"=w5, "NaN Color"=w4) -> (w2:T3)
  n45 = Merge Errors(w65, w68, w23, w89, w88, w87, w86, w85, w19, w42, w33, w34, w8, w10) -> (w90:errorcluster)
  n46 = call "AlliGator Laser Period.vi"() -> ("Laser Period"=w30:dbl[unit])
  n47 = call "AlliGator SYNC Period.vi"() -> ("SYNC Period"=w29:dbl[unit])
  n48 = call "AlliGator Number of Gates.vi"() -> ("# Gates"=w26:u32)
  n49 = call "AlliGator Nanotime Gate Separation.vi"() -> ("Nanotime Gate Separation"=w28:dbl[unit])
  n50 = Bundle By Name(cluster=T5 {"Laser Period"=0.0, "SYNC Period"=0.0, "# Gates"=0, "Gate Separation"=0.0} ("Data Information"), "Laser Period"=w30, "SYNC Period"=w29, "# Gates"=w26, "Gate Separation"=w28) -> (w27:T5)
  n51 = in-place {
    in-place-border: w119 -> [w160]
    in-place-border: w114 -> [w159]
    in-place-border: w113 -> [w158]
    in-place-border: w110 -> [w157]
    in-place-border: [w156] -> w109
    in-place-border: [w155] -> w106
    in-place-border: "Source Image Display" -> [w154]
    in-place-border: w104 -> [w153]
    in-place-border: w101 -> [w152]
    in-place-border: w95 -> [w151]
    in-place-border: w18 -> [w150]
    in-place-border: w90 -> [w149]
    in-place-border: [w148] -> w84
    in-place-border: [w147] -> w80
    in-place-border: w61 -> [w144]
    in-place-border: w55 -> [w143]
    in-place-border: w54 -> [w142]
    in-place-border: w53 -> [w141]
    in-place-border: w51 -> [w140]
    in-place-border: w50 -> [w139]
    in-place-border: w49 -> [w138]
    in-place-border: w43 -> [w137]
    in-place-border: w38 -> [w136]
    in-place-border: w37 -> [w135]
    in-place-border: w32 -> [w134]
    in-place-border: w32 -> [w133]
    in-place-border: w27 -> [w132]
    in-place-border: w22 -> [w131]
    in-place-border: w2 -> [w130]
    n52 = in-place-dvr #1("AlliGator IV DVR in") -> (w146:T17)  [unwired: 1 out]
    n53 = in-place {
      in-place-border: w160 -> [w229]
      in-place-border: w159 -> [w228]
      in-place-border: w158 -> [w227]
      in-place-border: w157 -> [w226]
      in-place-border: [w225] -> w156
      in-place-border: [w224] -> w155
      in-place-border: w154 -> [w223]
      in-place-border: w153 -> [w222]
      in-place-border: w152 -> [w221]
      in-place-border: w151 -> [w220]
      in-place-border: w150 -> [w219]
      in-place-border: w149 -> [w172]
      in-place-border: [w218] -> w148
      in-place-border: [w205] -> w147
      in-place-border: w144 -> [w206]
      in-place-border: w143 -> [w204]
      in-place-border: w142 -> [w203]
      in-place-border: w141 -> [w202]
      in-place-border: w140 -> [w178]
      in-place-border: w139 -> [w201]
      in-place-border: w138 -> [w200]
      in-place-border: w137 -> [w197]
      in-place-border: w136 -> [w189]
      in-place-border: w135 -> [w188]
      in-place-border: w134 -> [w180]
      in-place-border: w133 -> [w181]
      in-place-border: w132 -> [w174]
      in-place-border: w131 -> [w162]
      in-place-border: w130 -> [w161]
      # "used to be [[Sum Image]]"
      # "parse formula only once"
      # "1. Gets a temp image to\nbuild the overlay"
      n54 = in-place-cluster #2(w146) -> ("[[CSG Phasors]]"=w208:csg[][], "[[Valid Pixel?]]"=w207:bool[][], "Displayed Image"=w170:T1)  [unwired: 5 out]
      n55 = call "Alligator Variables Storage.vi"("AlliGator Variable"=AlliGator_Variables_List."X_Source Image:Palette Information" ("Alligator Variable"), "Error In"=w172) -> ("Error Out"=w195:errorcluster, "Data out"=w194:variant)  [unwired: 7 in, 1 out]
      n56 = Variant To Data(error in=w195, type=T10 {"Palette Name [# Colors,int?,inv?]"="", "Palette Type"=0, "Palette Colors"=[], "Interpolate?"=FALSE} ("Image Display Palette Information"), Variant=w194) -> (data=w192:T10, error out=w190:errorcluster)
      n57 = Bundle By Name(cluster=cluster{"Min Value":dbl, "Max Value":dbl} {"Min Value"=nan, "Max Value"=nan} ("Image Display Range"), "Max Value"=w189, "Min Value"=w188) -> (w163:cluster{"Min Value":dbl, "Max Value":dbl})
      n58 = call "IMAQ ImageToArray"("error in (no error)"=w172, "Image"=w170) -> ("Image Pixels (Float)"=w173:sgl[][], "error out"=w171:errorcluster)  [unwired: 2 in, 3 out]
      n59 = call "Image Display Get Pixel Color Information.vi"("Error In"=w190, "Image Display Range"=w163, "Image Display Palette Information"=w192) -> ("Error Out"=w185:errorcluster, "Image Scale Factor (256 colors)"=w186:sgl, "1D Color Array"=w187:cluster{"Red":u8, "Green":u8, "Blue":u8}[])  [unwired: 5 in, 1 out]
      n60 = call "IMAQ IntegerToColorValue"("error in (no error)"=w185, "U32 value"=w227) -> ("error out"=w183:errorcluster, "Color Value"=w216:T15)  [unwired: 3 in, 2 out]
      n61 = call "IMAQ IntegerToColorValue"("error in (no error)"=w185, "U32 value"=w228) -> ("error out"=w184:errorcluster, "Color Value"=w217:T15)  [unwired: 3 in, 2 out]
      n62 = call "Create Same Type Image.vi"("error in (no error)"=w172, "Name in"="TempPhasorRatioMapOverlay", "Image Src"=w223) -> ("error out"=w212:errorcluster, "Image Dst"=w214:T1)  [unwired: 6 in, 1 out]
      n63 = call "IMAQ Clear Overlay"("error in (no error)"=w212, "Image"=w214) -> ("error out"=w211:errorcluster, "Image Out"=w213:T1)  [unwired: 8 in]
      n64 = call <vilib>:"Clear Errors.vi"("error in (no error)"=w211, "specific error code to clear (0: all)"=w222) -> ("error out"=w210:errorcluster)  [unwired: 4 in, 1 out]
      n65 = Merge Errors(w171, w210, w184, w183) -> (w177:errorcluster)
      n66 = case shown="\"User-Defined Quantity\"" w178 {
        tunnel: w180 -> [_ w457]
        tunnel: [w452 w456] -> w176
        tunnel: w177 -> [w452 w453]
        frame "Phasor Ratio (f1 or a1)", Default {
        }
        frame "User-Defined Quantity" {
          n67 = call "AlliGator Computer User-defined Quantity.vi"("Init (F)"=TRUE, "Error In"=w453, "Formula"=w457, "Basic Quantities"=sgl[] []) -> ("Error Out"=w456:errorcluster)  [unwired: 6 in, 1 out]
        }
      }
      n68 = call "High Resolution Timing.vi"("Error In"=w176) -> ("relative seconds"=w215:dbl, "Error Out"=w175:errorcluster)  [unwired: 16 in, 1 out]
      n69 = call "AlliGator Phasor Frequency.vi"() -> ("Phasor Frequency"=w179:dbl[unit])
      n70 = call "Logical Processors Used.vi"() -> ("# Logical Processor Used"=w168:i32)  [unwired: 6 in]
      n71 = for "For Loop on V lines" {
        tunnel: w208 -> [w265] mode=indexing
        tunnel: w217 -> [w264]
        tunnel: w216 -> [w263]
        tunnel: w229 -> [w262]
        tunnel: w226 -> [w261]
        tunnel: w215 -> [w259]
        tunnel: [w259] -> w218
        tunnel: w221 -> [w258]
        tunnel: w220 -> [w257]
        tunnel: w219 -> [w231]
        tunnel: w213 -> [w268]
        tunnel: [w266] -> w166
        tunnel: [w256] -> w225 mode=indexing
        tunnel: w177 -> [w267]
        tunnel: [w255] -> w169 mode=concatenating
        tunnel: w207 -> [w254] mode=indexing
        tunnel: w206 -> [w253]
        tunnel: [w252] -> w199 mode=indexing
        tunnel: w204 -> [w251]
        tunnel: w203 -> [w250]
        tunnel: w202 -> [w249]
        tunnel: w178 -> [w248]
        tunnel: w201 -> [w247]
        tunnel: w200 -> [w246]
        tunnel: w197 -> [w245]
        tunnel: [w244] -> w198 mode=indexing
        tunnel: w173 -> [w243]
        workers-P: w168 -> [_]
        tunnel: w187 -> [w242]
        tunnel: w186 -> [w241]
        tunnel: [w240] -> w165 mode=indexing
        tunnel: [w239] -> w164
        tunnel: w180 -> [w238]
        tunnel: [w237] -> w182 mode=indexing
        tunnel: w175 -> [w236]
        tunnel: w179 -> [w235]
        tunnel: w174 -> [w234]
        tunnel: w163 -> [w233]
        tunnel: w162 -> [w232]
        tunnel: w161 -> [w230]
        i -> [w269]
        w239 = "Phasor Ratio Map Overlay" ("Group")
        # "y"
        n72 = for "For Loop on H columns" {
          tunnel: w269 -> [w299]
          tunnel: w239 -> [w308]
          tunnel: w265 -> [w303] mode=indexing
          tunnel: w264 -> [w302]
          tunnel: w263 -> [w301]
          tunnel: w262 -> [w304]
          tunnel: w261 -> [w300]
          tunnel: w258 -> [w297]
          tunnel: w257 -> [w296]
          tunnel: w268 -> [w309]
          tunnel: [w306] -> w266
          tunnel: w267 -> [w307]
          tunnel: [w305] -> w255 mode=indexing
          tunnel: [w294] -> w260 mode=indexing if=w295
          tunnel: w254 -> [w292] mode=indexing
          tunnel: w253 -> [w293]
          tunnel: [w291] -> w252 mode=indexing
          tunnel: w251 -> [w290]
          tunnel: w250 -> [w289]
          tunnel: w249 -> [w288]
          tunnel: w248 -> [w287]
          tunnel: w247 -> [w286]
          tunnel: w246 -> [w285]
          tunnel: w245 -> [w284]
          tunnel: [w283] -> w244 mode=indexing
          tunnel: w243 -> [w282]
          tunnel: w242 -> [w281]
          tunnel: w241 -> [w280]
          tunnel: [w279] -> w240 mode=indexing
          tunnel: w238 -> [w278]
          tunnel: [w277] -> w237 mode=indexing
          tunnel: w236 -> [w276]
          tunnel: w235 -> [w275]
          tunnel: w234 -> [w274]
          tunnel: w233 -> [w273]
          tunnel: w232 -> [w272]
          tunnel: w231 -> [w271]
          tunnel: w230 -> [w270]
          i -> [w298]
          # "x"
          n73 = case shown="True" w292 {
            tunnel: w309 -> [w313 w359]
            tunnel: w308 -> [_ w358]
            tunnel: w307 -> [w312 w357]
            tunnel: [w313 w355] -> w306
            tunnel: [w312 w354] -> w305
            tunnel: w304 -> [_ w352]
            tunnel: w303 -> [_ w326]
            tunnel: w302 -> [_ w351]
            tunnel: w301 -> [_ w350]
            tunnel: w300 -> [_ w349]
            tunnel: w299 -> [_ w340]
            tunnel: w298 -> [_ w341]
            tunnel: w297 -> [_ w348]
            tunnel: w296 -> [_ w347]
            tunnel: [_ w345] -> w295
            tunnel: [_ 1] -> w294
            tunnel: w293 -> [_ w343]
            tunnel: [w310 w325] -> w291
            tunnel: w290 -> [_ w339]
            tunnel: w289 -> [_ w328]
            tunnel: w288 -> [_ w338]
            tunnel: w287 -> [_ w337]
            tunnel: w286 -> [_ w332]
            tunnel: w285 -> [_ w331]
            tunnel: w284 -> [_ w333]
            tunnel: [w310 w324] -> w283
            tunnel: w282 -> [_ w336]
            tunnel: w281 -> [_ w322]
            tunnel: w280 -> [_ w335]
            tunnel: [u32 16777216 ("Reference 1") w334] -> w279
            tunnel: w278 -> [_ w330]
            tunnel: [w310 w314] -> w277
            tunnel: w276 -> [_ w329]
            tunnel: w275 -> [_ w327]
            tunnel: w274 -> [_ w320]
            tunnel: w273 -> [_ w318]
            tunnel: w272 -> [_ w317]
            tunnel: w271 -> [_ w316]
            tunnel: w270 -> [_ w315]
            frame False {
              w310 = sgl nan
            }
            frame True {
              n74 = call "Phasor Get Phasor Ratio.vi"("z"=w326, "Error In"=w329, "Reference Phasor 2"=w338, "Reference Phasor 1"=w328) -> ("Error Out"=w323:errorcluster, "Phasor Ratio (f1)"=w325:dbl)  [unwired: 5 in, 1 out]
              n75 = case shown="\"Average Lifetime (<tau>_i or <tau>_a))\"" w337 {
                tunnel: [w399 w406 w426] -> w314
                tunnel: w333 -> [w400 w407 w420]
                tunnel: w332 -> [w403 w410 w417]
                tunnel: w331 -> [w402 w409 w416]
                tunnel: w325 -> [w401 w408 w418]
                tunnel: w330 -> [_ _ w425]
                tunnel: w323 -> [w396 w405 w414]
                tunnel: w327 -> [_ _ w419]
                tunnel: w326 -> [_ _ w415]
                tunnel: [w397 w406 w423] -> w324
                tunnel: [w395 w404 w413] -> w321
                tunnel: w320 -> [_ _ w412]
                frame "Phasor Ratio (f1 or a1)", Default {
                  # "f1 or a1 depending on average lifetime option"
                  n76 = call "Phasor Convert Ratio to Amplitude Ratio & Average Lifetime.vi"("Compute Amplitude Ratio"=w400, "error in (no error)"=w396, "Reference Lifetime 2"=w402, "Reference Lifetime 1"=w403, "Phasor Ratio (f1)"=w401) -> ("error out"=w395:errorcluster, "Average Lifetime"=w398:dbl[unit], "Phasor/Amplitude Ratio"=w399:dbl)  [unwired: 2 in, 2 out]
                  n77 = node(w398) -> (w397:dbl)
                }
                frame "Average Lifetime (<tau>_i or <tau>_a))" {
                  # "<tau>_i or <tau>_a depending on average lifetime option"
                  n78 = call "Phasor Convert Ratio to Amplitude Ratio & Average Lifetime.vi"("Compute Amplitude Ratio"=w407, "error in (no error)"=w405, "Reference Lifetime 2"=w409, "Reference Lifetime 1"=w410, "Phasor Ratio (f1)"=w408) -> ("error out"=w404:errorcluster, "Average Lifetime"=w411:dbl[unit])  [unwired: 2 in, 3 out]
                  n79 = node(w411) -> (w406:dbl)
                }
                frame "User-Defined Quantity" {
                  n80 = call "AlliGator Compute Basic Quantities.vi"("Phasor Ratio (f1)"=w418, "Data Information"=w412, "Reference Lifetime 1"=w417, "Reference Lifetime 2"=w416, "Complex Phasor"=w415, "error in (no error)"=w414, "Phasor Frequency"=w419, "Compute Amplitude Ratio"=w420) -> ("Average Lifetime"=w423:dbl, "Basic Quantities"=w422:dbl[], "error out"=w421:errorcluster)  [unwired: 5 in]
                  n81 = call "AlliGator Computer User-defined Quantity.vi"("Init (F)"=FALSE, "Error In"=w421, "Formula"=w425, "Basic Quantities"=w422) -> ("Error Out"=w413:errorcluster, "User-defined Quantity"=w426:sgl)  [unwired: 6 in]
                }
              }
              n82 = Bundle By Name(cluster=w343, "Complex Phasor"=w326, "Phasor Ratio"=w325, "Mapped Quantity"=w314) -> (w342:T8)
              n83 = case shown="\"Use Custom Map\"" w347 {
                tunnel: w352 -> [w432 w449]
                tunnel: [w436 w437] -> w353
                tunnel: w351 -> [w431 _]
                tunnel: w350 -> [w430 _]
                tunnel: [w435 w451] -> w346
                tunnel: w349 -> [w433 w448]
                tunnel: w316 -> [_ w446]
                tunnel: w342 -> [w434 w450]
                tunnel: w339 -> [w429 w442]
                tunnel: w321 -> [w428 w440]
                tunnel: [w427 w447] -> w319
                tunnel: w315 -> [_ w445]
                tunnel: w314 -> [_ w441]
                frame "Interpolate Reference Colors", Default {
                  n84 = call "AlliGator Get Phasor Ratio Interpolated Color v2.vi"("Color 2"=w430, "Color 1"=w431, "Color Fading?"=w433, "Error In"=w428, "Phasor Ratio/Average Lifetime Display Range"=w429, "-d_0"=w432, "Phasor Ratio Data"=w434) -> ("Error Out"=w427:errorcluster, "Transparent?"=w435:bool, "Overlay Color"=w436:T15)  [unwired: 2 in]
                }
                frame "Use Custom Map" {
                  n85 = Unbundle By Name(w442) -> ("Max"=w443:dbl, "Min"=w444:dbl)
                  n86 = call "Color Pixel with Color Scale.vi"("Color Scale 1D Color Array"=w446, "Limit+NaN Colors"=w445, "Error In"=w440, "Color Scale Min Value"=w444, "Color Scale Max Value"=w443, "Pixel Value"=w441) -> ("Error Out"=w438:errorcluster, "Pixel Color"=w439:T15)  [unwired: 4 in]
                  n87 = call "AlliGator Get Phasor Ratio Map Color v3.vi"("Color Fading?"=w448, "Error In"=w438, "Pixel Color"=w439, "-d_0"=w449, "Phasor Ratio Data"=w450) -> ("Error Out"=w447:errorcluster, "Transparent?"=w451:bool, "Overlay Color"=w437:T15)  [unwired: 4 in]
                }
              }
              n88 = case shown="False" w346 {
                tunnel: w359 -> [w373 w393]
                tunnel: w353 -> [w375 _]
                tunnel: w358 -> [_ _]
                tunnel: w357 -> [w374 w394]
                tunnel: [w364 w394] -> w356
                tunnel: [w369 w393] -> w355
                tunnel: w341 -> [w372 _]
                tunnel: w340 -> [w371 _]
                tunnel: w348 -> [w370 _]
                tunnel: w336 -> [w368 _]
                tunnel: w322 -> [w367 _]
                tunnel: w335 -> [w366 _]
                tunnel: [w365 u32 16777216 ("Reference 1")] -> w334
                tunnel: w319 -> [_ _]
                tunnel: w318 -> [w361 _]
                tunnel: w317 -> [w360 _]
                frame False {
                  # "Not transparent"
                  n89 = case shown="True" w370 {
                    tunnel: [w377 w385] -> w362
                    tunnel: w375 -> [w378 w382]
                    tunnel: [w378 w386] -> w363
                    tunnel: w374 -> [w377 w384]
                    tunnel: w373 -> [w376 w389]
                    tunnel: w372 -> [_ w391]
                    tunnel: w371 -> [_ w390]
                    tunnel: [w376 w389] -> w369
                    tunnel: w368 -> [_ w388]
                    tunnel: w367 -> [_ w383]
                    tunnel: w366 -> [_ w380]
                    tunnel: w361 -> [_ w381]
                    tunnel: w360 -> [_ w379]
                    frame False {
                      # "Display overlay color as is"
                    }
                    frame True {
                      # "Use Image Brightness"
                      n90 = Index Array(array=w388, index (row)=w390, index (col)=w391) -> (element=w387:sgl)
                      n91 = call "Blend Overlay Color with Background.vi"("Overlay Color Value"=w382, "Image Scale Factor"=w380, "Blend Overlay with Background"=w379, "error in (no error)"=w384, "Image Display Range"=w381, "Image Color Array"=w383, "Pixel Value"=w387) -> ("error out"=w385:errorcluster, "Scaled/Blended Overlay Color Value"=w386:T15)  [unwired: 3 in]
                    }
                  }
                  n92 = call "IMAQ ColorValueToInteger"("error in (no error)"=w362, "Color Value"=w363) -> ("error out"=w364:errorcluster, "U32 value"=w365:u32)  [unwired: 3 in, 2 out]
                }
                frame True {
                  # "Transparent overlay"
                }
              }
              n93 = Not(x=w346) -> (.not. x?=w345:bool)
              n94 = call "Tiny Clear Error.vi"("Error In"=w356) -> ("no Error Out"=w354:errorcluster)  [unwired: 8 in]
            }
          }
        }
        n95 = Add Array Elements(numeric array=w260) -> (sum=w256:i32)
      }
      n96 = Merge Errors(w169) -> (w167:errorcluster)
      n97 = call "IMAQ Overlay Bitmap"("Group"=w164, "error in (no error)"=w167, "Bitmap"=w165, "Image"=w166) -> ("error out"=w205:errorcluster, "Image Out"=w224:T1)  [unwired: 6 in]
      n98 = in-place-cluster #2("[[CSG Phasors]]"=w208, "[[Valid Pixel?]]"=w207, "[[Phasor Ratios]]"=w199, "[[Average Lifetimes]]"=w198, "[[User-defined Quantities]]"=w182, "User-defined Quantity"=w181, "Amplitude Weighted Average Lifetime"=w197, "Displayed Image"=w170) -> (w145:T17)
    }
    n99 = in-place-dvr #1(w145) -> (→"AlliGator IV DVR out":refnum<data-value>, w69:errorcluster)
  }
  n100 = Add Array Elements(numeric array=w109) -> (sum=→"# Overlay Pixels":i32)
  n101 = Merge Errors(w69, w80) -> (w75:errorcluster)
  n102 = call "High Resolution Timing.vi"("relative seconds (NaN)"=w84, "Error In"=w75) -> ("relative seconds"=w82:dbl, "elapsed (relative) seconds"=→"Overlay Compute (s)":dbl, "Error Out"=w81:errorcluster)  [unwired: 15 in]
  n103 = call "IMAQ Clear Overlay"("error in (no error)"=w81, "Image"="Source Image Display") -> ("error out"=w105:errorcluster, "Image Out"=w108:T1)  [unwired: 8 in]
  n104 = call <vilib>:"Clear Errors.vi"("error in (no error)"=w105, "specific error code to clear (0: all)"=w104) -> ("error out"=w74:errorcluster)  [unwired: 4 in, 1 out]
  n105 = call "High Resolution Timing.vi"("relative seconds (NaN)"=w82, "Error In"=w74) -> ("relative seconds"=w78:dbl, "elapsed (relative) seconds"=→"Overlay Erase (s)":dbl, "Error Out"=w73:errorcluster)  [unwired: 15 in]
  n106 = call "IMAQ Copy Overlay"("error in (no error)"=w73, "Image Dst"=w108, "Image Src"=w106) -> ("error out"=w72:errorcluster, "Image Dst Out"=→"Source Image Display out":T1)  [unwired: 7 in]
  n107 = call "High Resolution Timing.vi"("relative seconds (NaN)"=w78, "Error In"=w72) -> ("elapsed (relative) seconds"=→"Overlay Copy (s)":dbl, "Error Out"=→"Error Out":errorcluster)  [unwired: 15 in, 1 out]
